vi "Test Read.vi"() -> ()   [LabVIEW 2014, in "Arduino SoftwareSerial Wrapper.lvlib"]
uses:
  Arduino SoftwareSerial Wrapper.lvlib
panel:
  out "Bytes to read":u16
  out "Output char":u8
  out "Error Out":errorcluster
  in  "Error In":errorcluster
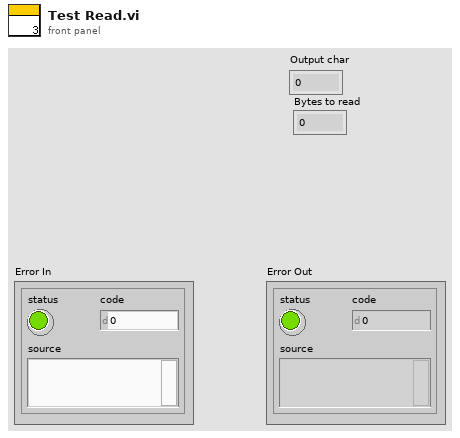
[diagram p1: front panel]
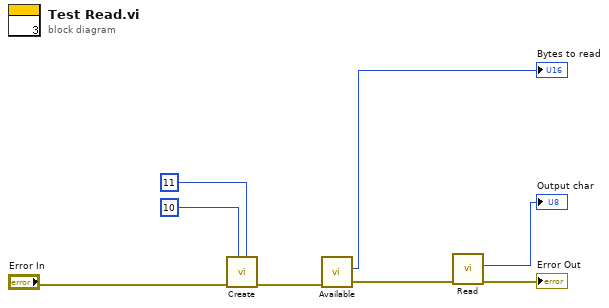
[diagram p0: block diagram]
diagram:
  n1 = call "Create.vi"("arduino RX pin"=u8 11 ("RX pin"), "arduino TX pin"=u8 10 ("RX pin"), "Error In"="Error In") -> ("Error Out"=w5:errorcluster)  [unwired: 8 in]
  n2 = call "Available.vi"("Error In"=w5) -> ("Error Out"=w3:errorcluster, "Bytes to read"=→"Bytes to read":u16)  [unwired: 9 in]
  n3 = call "Read.vi"("Error In"=w3) -> ("Error Out"=→"Error Out":errorcluster, "Output char"=→"Output char":u8)  [unwired: 9 in]
